vi "Queue-Push Element.vi"(8 "error in":errorcluster, 10 "element":variant, 11 "Buffer in":refnum<data-value>) -> (0 "error out":errorcluster, 1 "overflowed":bool, 2 "overflow":variant, 3 "Buffer":refnum<data-value>)   [LabVIEW 2013, in "CircularBuffer.lvlib" / "VariantBuffer.lvclass"]
doc: "This VI writes one data element into the current location in the buffer. The location in the buffer is updated automatically."
uses:
  VariantBuffer.lvclass
  buffer-errors -- ring.ctl
  VariantBuffer.lvclass/VariantBuffer.ctl
  buffer-event -- enum.ctl
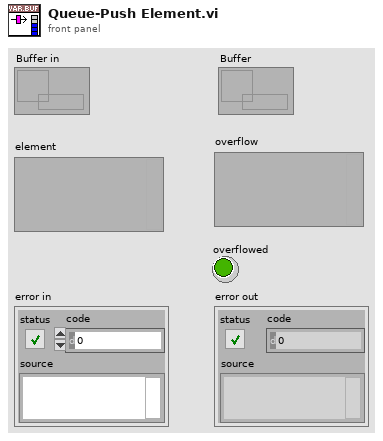
[diagram p1: front panel]
types:
  T1 = typedef "CircularBuffer.lvlib/VariantBuffer.lvclass/buffer-errors -- ring.ctl" = i32
  T2 = typedef "CircularBuffer.lvlib/VariantBuffer.lvclass/buffer-type -- enum.ctl" = enum16{"Queue", "Stack"}
  T3 = typedef "CircularBuffer.lvlib/VariantBuffer.lvclass/buffer-event -- enum.ctl" = enum16{"element-added", "element-removed", "filled", "emptied", "resized", "default-changed", "destroyed"}
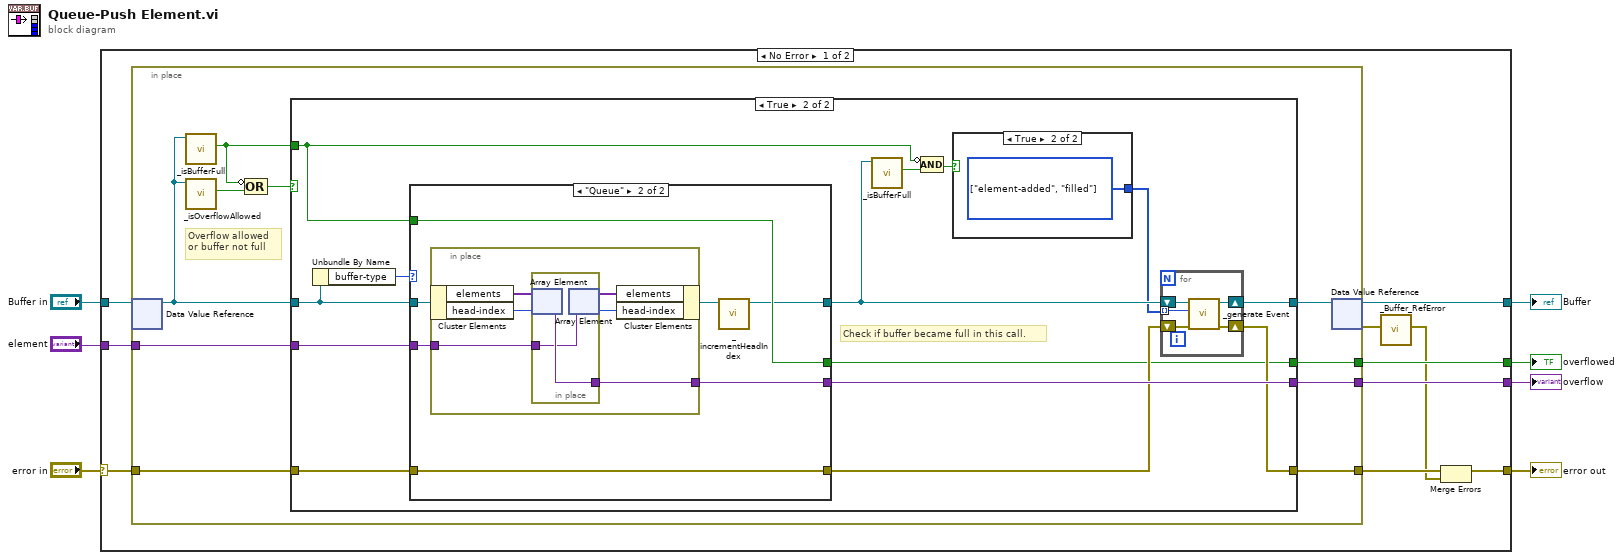
[diagram p0: block diagram]
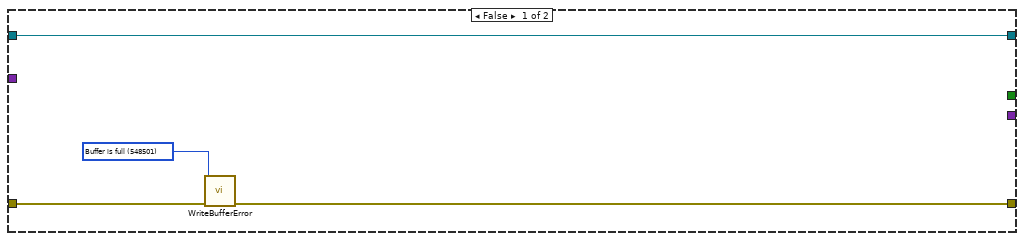
[diagram p2: hidden frame]
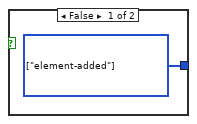
[diagram p3: hidden frame]
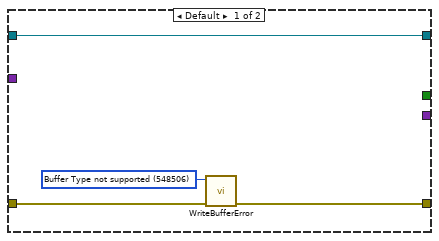
[diagram p4: hidden frame]
diagram:
  n1 = case shown="No Error" "error in" {
    selector: "error in" -> [w11 w73]
    tunnel: "Buffer in" -> [w17 w72]
    tunnel: [w14 w72] -> w6
    tunnel: [w16 w73] -> w5
    tunnel: "element" -> [w15 _]
    tunnel: [w13 _] -> w2
    tunnel: [w12 _] -> w1
    frame No Error {
      n2 = in-place {
        in-place-border: w15 -> [w27]
        in-place-border: [w26] -> w13
        in-place-border: [w25] -> w12
        in-place-border: w11 -> [w21]
        in-place-border: [w20] -> w10
        # "Overflow allowed\nor buffer not full"
        n3 = in-place-dvr #1(w17) -> (w24:refnum<class "VariantBuffer.lvclass">)  [unwired: 1 out]
        n4 = call "_isBufferFull.vi"("VariantBuffer in"=w24) -> ("isFull"=w19:bool)  [unwired: 10 in]
        n5 = call "_isOverflowAllowed.vi"("VariantBuffer in"=w24) -> ("Allow Overflow?"=w18:bool)  [unwired: 10 in]
        n6 = Compound Arithmetic op=OR(invert w19, w18) -> (w23:bool)
        n7 = case shown="True" w23 {
          tunnel: w27 -> [_ w45]
          tunnel: [w29 w40] -> w22
          tunnel: [_ w44] -> w26
          tunnel: [_ w32] -> w25
          tunnel: w24 -> [w29 w43]
          tunnel: w21 -> [w31 w41]
          tunnel: [w30 w39] -> w20
          tunnel: w19 -> [_ w33]
          frame False {
            w28 = T1 548501 items=["No error"=0, "Generic Buffer error"=548500, "Buffer is full"=548501, "Buffer is empty"=548502, "Buffer size cannot be 0"=548503, "Buffer reference is invalid"=548504, "Buffer event reference invalid"=548505] ("buffer-errors")
            n8 = call "WriteBufferError.vi"("error in (no error)"=w31, "buffer-errors"=w28) -> ("error out"=w30:errorcluster)  [unwired: 9 in]
          }
          frame True {
            # "Check if buffer became full in this call."
            n9 = Unbundle By Name(w43) -> ("buffer-type"=w42:T2)
            n10 = case shown="\"Queue\"" w42 {
              tunnel: w45 -> [_ w63]
              tunnel: [_ w62] -> w44
              tunnel: [_ w59] -> w32
              tunnel: w43 -> [w56 w61]
              tunnel: [w56 w57] -> w37
              tunnel: [w54 w60] -> w38
              tunnel: w41 -> [w55 w60]
              tunnel: w33 -> [_ w59]
              frame Default {
                w53 = T1 548506 items=["No error"=0, "Generic Buffer error"=548500, "Buffer is full"=548501, "Buffer is empty"=548502, "Buffer size cannot be 0"=548503, "Buffer reference is invalid"=548504, "Buffer event reference invalid"=548505, "Buffer Type not supported"=548506] ("buffer-errors")
                n11 = call "WriteBufferError.vi"("error in (no error)"=w55, "buffer-errors"=w53) -> ("error out"=w54:errorcluster)  [unwired: 9 in]
              }
              frame "Queue" {
                n12 = in-place {
                  in-place-border: w63 -> [w68]
                  in-place-border: [w65] -> w62
                  n13 = in-place-cluster #2(w61) -> ("elements"=w69:variant[], "head-index"=w66:i32)
                  n14 = in-place {
                    in-place-border: w68 -> [w70]
                    in-place-border: [w71] -> w65
                    n15 = in-place-array #3(w69, w66) -> (w71:variant)
                    n16 = in-place-array #3(w70) -> (w67:variant[], w64:i32)
                  }
                  n17 = in-place-cluster #2("elements"=w67, "head-index"=w64) -> (w58:refnum<class "VariantBuffer.lvclass">)
                }
                n18 = call "_incrementHeadIndex.vi"("VariantBuffer in"=w58) -> ("VariantBuffer out"=w57:refnum<class "VariantBuffer.lvclass">)  [unwired: 10 in]
              }
            }
            n19 = call "_isBufferFull.vi"("VariantBuffer in"=w37) -> ("isFull"=w36:bool)  [unwired: 10 in]
            n20 = Compound Arithmetic op=AND(invert w33, w36) -> (w35:bool)
            n21 = case shown="True" w35 {
              tunnel: [w46 w47] -> w34
              frame False {
                w46 = T3[] [enum."element-added"] items=["element-added", "element-removed", "filled", "emptied", "resized", "default-changed", "destroyed"]
              }
              frame True {
                w47 = T3[] [enum."element-added", enum."filled"] items=["element-added", "element-removed", "filled", "emptied", "resized", "default-changed", "destroyed"]
              }
            }
            n22 = for {
              tunnel: w34 -> [w50] mode=indexing
              shift-right: [w52] -> w40
              shift-left: w37 -> [w51]
              shift-right: [w49] -> w39
              shift-left: w38 -> [w48]
              n23 = call "_generate Event.vi"("error in"=w48, "event"=w50, "VariantBuffer"=w51) -> ("error out"=w49:errorcluster, "VariantBuffer out"=w52:refnum<class "VariantBuffer.lvclass">)  [unwired: 7 in]
            }
          }
        }
        n24 = in-place-dvr #1(w22) -> (w14:refnum<data-value>, w9:errorcluster)
      }
      n25 = call "_Buffer_RefError.vi"("error in (no error)"=w9) -> ("error out"=w8:errorcluster)  [unwired: 10 in]
      n26 = Merge Errors(w10, w8) -> (w16:errorcluster)
    }
    frame Error {
    }
  }
  "error out" <- w5
  "Buffer" <- w6
  "overflow" <- w2
  "overflowed" <- w1
